vi "Day08-create_set.vi"(11 "sorted array":u8[](array[numeric])) -> (3 "Set":set{u8}(c389))   [LabVIEW 2021]
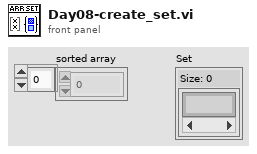
[diagram p1: front panel]
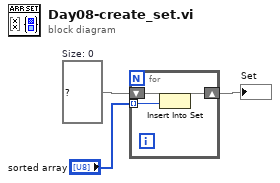
[diagram p0: block diagram]
diagram:
  w2 = set{u8} {}  # Size: 0
  n1 = for {
    tunnel: "sorted array" -> [w6] mode=indexing
    shift-right: [w5] -> w3
    shift-left: w2 -> [w4]
    n2 = Insert Into Set(10:w6, 11:w4) -> (3:w5:set{u8})  [unwired: 1 out]
  }
  "Set" <- w3
